vi "S2Alarm.vi"(8 "error in":errorcluster, 11 "HasAlarm":bool) -> (0 "error out":errorcluster)   [LabVIEW 2018, in "GUI.lvclass"]
uses:
  GUI.lvclass
  Queue/Queue Data.ctl
  Queue/State.ctl
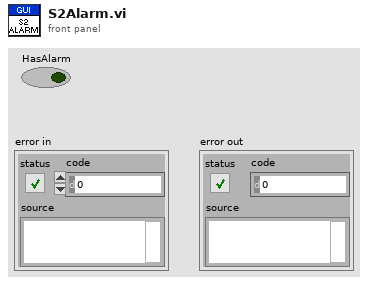
[diagram p1: front panel]
types:
  T1 = typedef "GUI.lvclass/Queue Data.ctl" = cluster{"State":T2, "Data":variant}
  T2 = typedef "GUI.lvclass/State.ctl" = enum16{"Initialize", "LoadConfig", "SaveConfig", "S1Alarm", "S2Alarm", "S1EndOfTest", "S2EndOfTest", "Monitor", "Error", "Exit"}
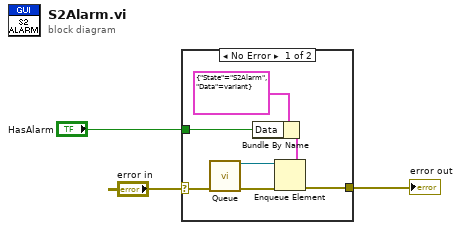
[diagram p0: block diagram]
diagram:
  n1 = case shown="No Error" "error in" {
    selector: "error in" -> [w10 w11]
    tunnel: [w7 w11] -> w3
    tunnel: "HasAlarm" -> [w4 _]
    frame No Error {
      n2 = call "Queue.vi"("error in"=w10) -> ("error out"=w9:errorcluster, "queue out"=w8:refnum<queue>)  [unwired: 9 in]
      n3 = Bundle By Name(cluster=T1 {"State"=enum."S2Alarm", "Data"=variant} ("element"), "Data"=w4) -> (w5:T1)
      n4 = Enqueue Element(queue=w8, element=w5, error in (no error)=w9) -> (error out=w7:errorcluster)  [unwired: 1 in, 2 out]
    }
    frame Error {
    }
  }
  "error out" <- w3
